vi "Handle Error.vi"(8 "error in (no error)":errorcluster, 11 "RP Communicator in":refnum<class "RP Communicator.lvclass">) -> (0 "error out":errorcluster, 3 "RP Communicator out":refnum<class "RP Communicator.lvclass">)   [LabVIEW 2024, in "RP Communicator.lvclass"]
uses:
  RP Communicator.lvclass
panel:
  out "call chain":string[](array[string])
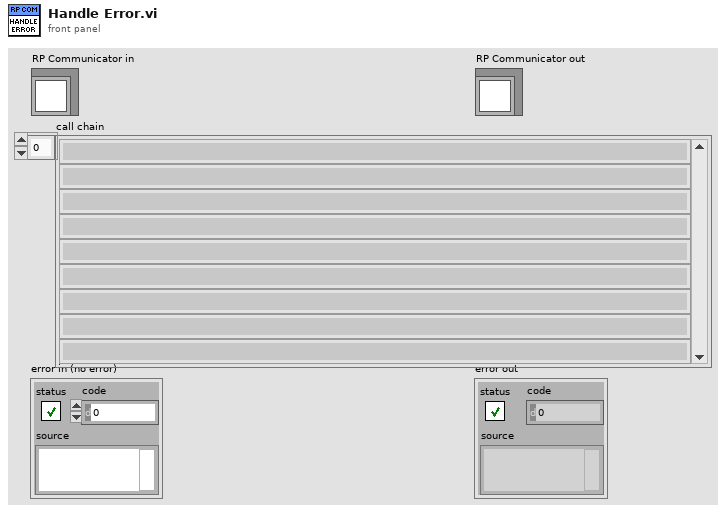
[diagram p1: front panel]
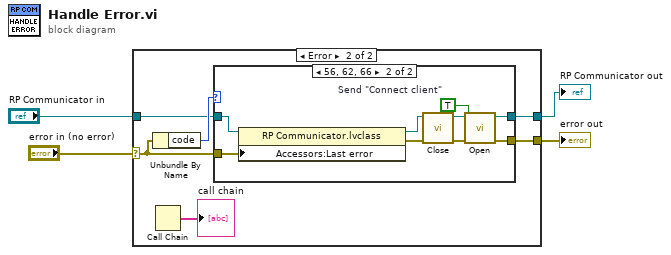
[diagram p0: block diagram]
diagram:
  n1 = case shown="Error" "error in (no error)" {
    selector: "error in (no error)" -> [w5 w11]
    tunnel: [w5 w10] -> w3
    tunnel: [w6 w9] -> w1
    tunnel: "RP Communicator in" -> [w6 w8]
    frame No Error {
    }
    frame Error {
      n2 = Unbundle By Name(w11) -> ("code"=w12:i32)
      n3 = Call Chain() -> (call chain=→"call chain":string[])
      n4 = case shown="56, 62, 66" w12 {
        tunnel: w11 -> [w14 w21]
        tunnel: [w14 w16] -> w10
        tunnel: w8 -> [w13 w19]
        tunnel: [w13 w17] -> w9
        frame 0, Default {
        }
        frame 56, 62, 66 {
          w15 = TRUE  # Send "Connect client"
          n5 = property class="RP Communicator.lvclass"(reference=w19, "Accessors:Last error"=w21) -> (reference out=w18:refnum<class "RP Communicator.lvclass">, error out=w20:errorcluster)  [unwired: 1 in]
          n6 = call-dynamic "Close.vi"("error in (no error)"=w20, "RP Communicator in"=w18) -> ("error out"=w23:errorcluster, "RP Communicator out"=w22:refnum<class "RP Communicator.lvclass">)  [unwired: 8 in]
          n7 = call-dynamic "Open.vi"("error in (no error)"=w23, "Send \"Connect client\""=w15, "RP Communicator in"=w22) -> ("error out"=w16:errorcluster, "RP Communicator out"=w17:refnum<class "RP Communicator.lvclass">)  [unwired: 7 in]
        }
      }
    }
  }
  "error out" <- w3
  "RP Communicator out" <- w1
